vi "New Three.vi"() -> ()   [LabVIEW 2015]
doc: "This example VI shows how to convert string data elements to numeric elements so it can be graphed and displayed on an XY Graph."
uses:
  <instrlib>/Keithley 27XX/Public/Configure/Measurement Specific/Configure Thermocouple.vi
  <instrlib>/Keithley 27XX/Keithley 27XX.lvlib
panel:
  out "Voltage 2":dbl(graph)
  out "Voltage 1":dbl(graph)
  out "Temperature Ch 1":dbl(graph)
  out "Temperature Ch 2":dbl(graph)
  out "appended array":dbl[](array[numeric])
  out "Iteration":i32
  out "x-y":dbl
  in  "Pause/Continue":bool
  out "error out 2425":errorcluster
  in  "range":i32
  in  "function":i32(slide)
  in  "error in (no error) 2":errorcluster
  in  "reset device":u16(slide)=1
  in  "id query":u16(slide)=1
  in  "resource name":string="GPIB0::20::INSTR"
  out "Temp Ch 4":dbl
  out "Temp Ch 3":dbl
  out "Temp Ch 2":dbl
  out "Temp Ch 1":dbl
  out "Voltage Ch 1":dbl
  out "Voltage Ch 2":dbl
  in  "stop":bool
  in  "Number of channels 2":i32=2
  in  "Function (0: DC Voltage)":u16(ring) items=["DC Voltage", "AC Voltage", "DC Current", "AC Current", "Resistance", "Four-Wire Resistance", "Temperature (C)", "Frequency", "Period", "Continuity"]
  in  "Channel List (101) 2":string="101:102"
  in  "Serial Configuration 2":T1={"Baud Rate (9600)"=9600, "Flow Control (1: XON/XOFF)"=1, "Termination Char (0:CR)"=0} {"Termination Char (0:CR)" items=["CR", "LF", "CRLF (Do not use)", "LFCR (Do not use)"]; "Flow Control (1: XON/XOFF)" items=["None", "XON/XOFF", "RTS/CTS (2701 Only)", "XON/XOFF & RTS/CTS (2701 Only)"]; "Baud Rate (9600)" items=["300"=300, "600"=600, "1200"=1200, "2400"=2400, "4800"=4800, "9600"=9600, "19.2k"=19200, "38.4k (2701 Only)"=38400, "57.6k (2701 Only)"=57600, "115.2k (2701 Only)"=115200]}
  in  "Keithley VISA resource name 2":refnum<visa-resource-name>="GPIB0::19::INSTR"
  in  "Enable Open Detector? (False)":bool=TRUE
  in  "Simulated Reference Temperature (23 deg C)":dbl=23.0
  in  "Reference Junction Type (1: Internal)":u16(ring)=1 items=["Simulated", "Internal", "External"]
  in  "Thermocouple Type (1: K)":u16(ring)=1 items=["J", "K", "T", "E", "R", "S", "B", "N"]
  in  "Number of channels":i32=4
  in  "Function (6: Temp)":u16(ring)=6 items=["DC Voltage", "AC Voltage", "DC Current", "AC Current", "Resistance", "Four-Wire Resistance", "Temperature (C)", "Frequency", "Period", "Continuity"]
  in  "Channel List (101)":string="101"
  in  "Serial Configuration":T1={"Baud Rate (9600)"=9600, "Flow Control (1: XON/XOFF)"=1, "Termination Char (0:CR)"=0} {"Termination Char (0:CR)" items=["CR", "LF", "CRLF (Do not use)", "LFCR (Do not use)"]; "Flow Control (1: XON/XOFF)" items=["None", "XON/XOFF", "RTS/CTS (2701 Only)", "XON/XOFF & RTS/CTS (2701 Only)"]; "Baud Rate (9600)" items=["300"=300, "600"=600, "1200"=1200, "2400"=2400, "4800"=4800, "9600"=9600, "19.2k"=19200, "38.4k (2701 Only)"=38400, "57.6k (2701 Only)"=57600, "115.2k (2701 Only)"=115200]}
  in  "Keithley VISA resource name":refnum<visa-resource-name>="GPIB0::19::INSTR"
  # "2700 Temp INIT"
  # "Keithley 2425 INIT"
  # "2700 Voltage INIT"
  # "File INIT"
  # "Operations"
  # "Only 4 Ch implemented"
  # "Data"
  # "Loop 1"
  # "Loop 2"
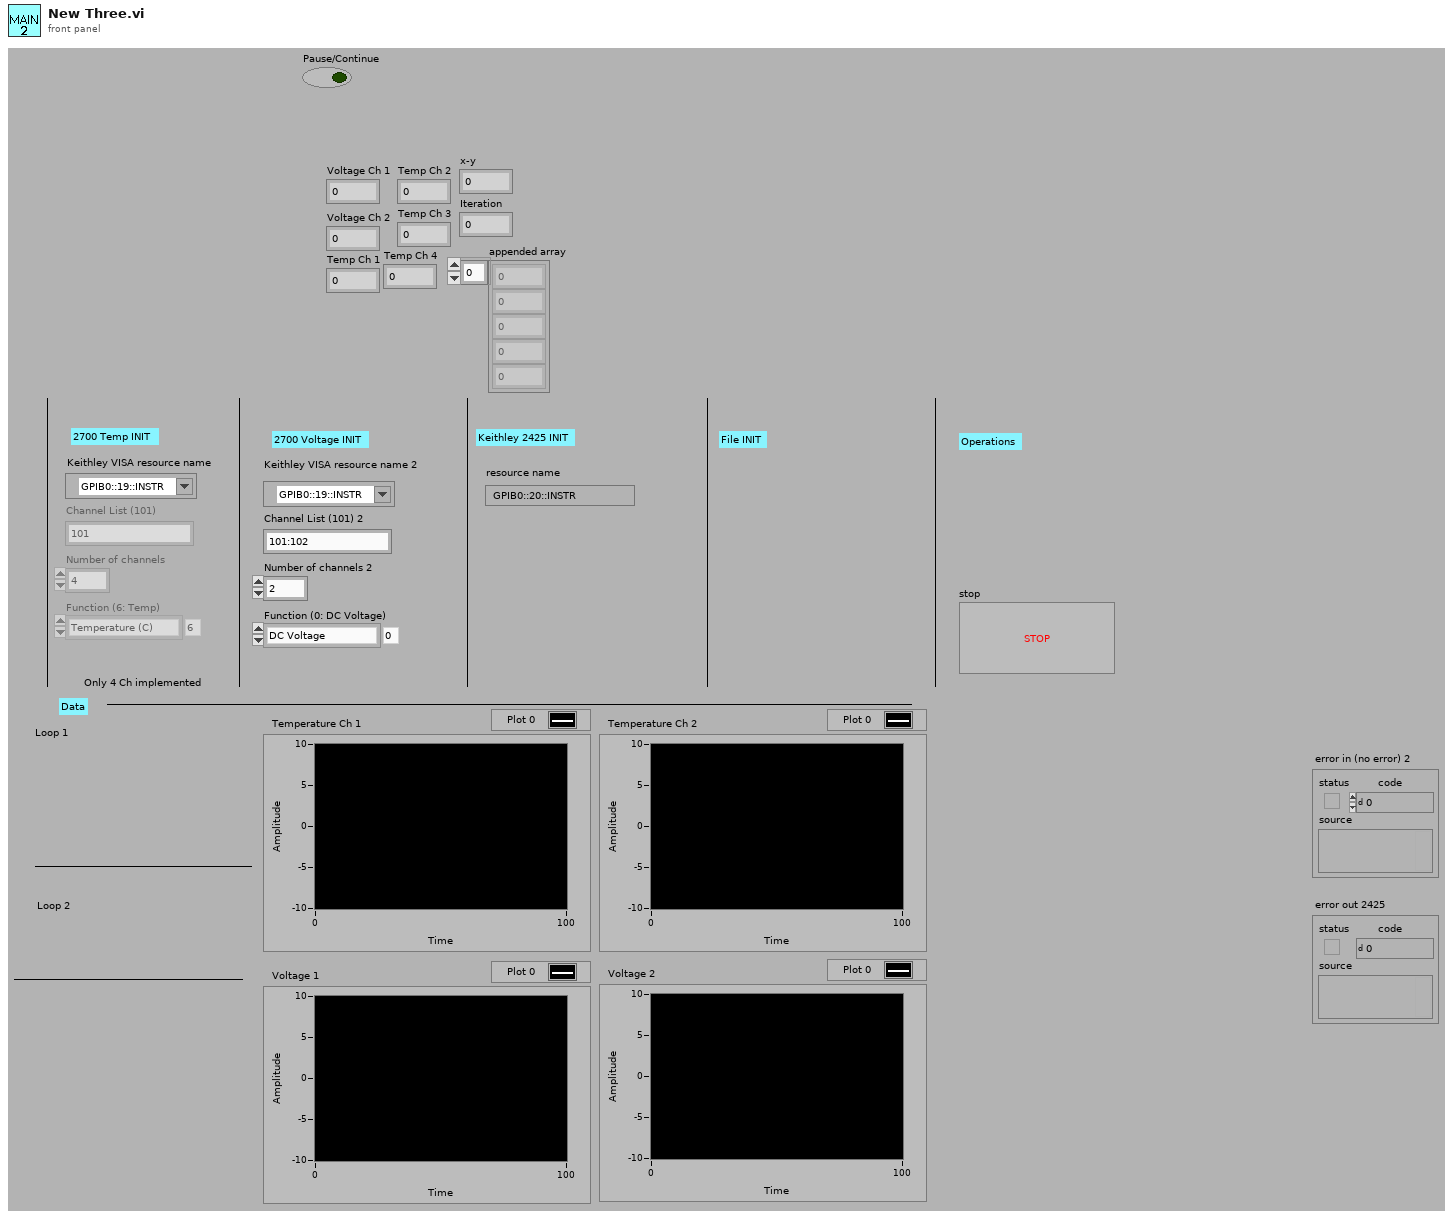
[diagram p1: front panel]
types:
  T1 = cluster{"Baud Rate (9600)":u32, "Flow Control (1: XON/XOFF)":u16, "Termination Char (0:CR)":u16}
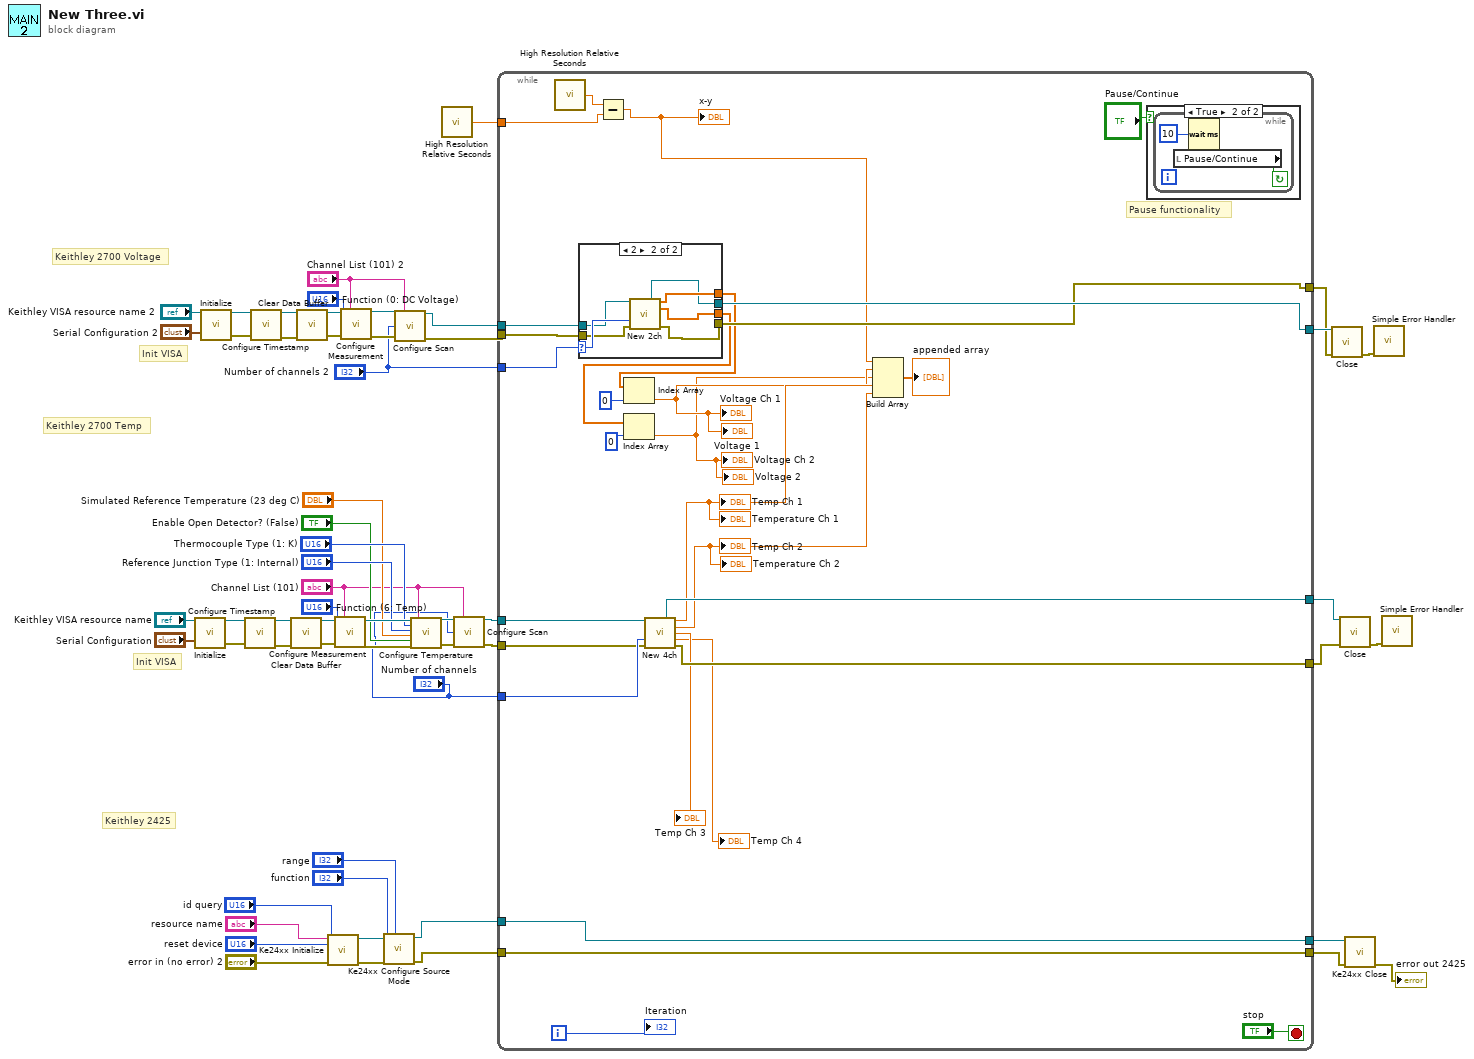
[diagram p0: block diagram]
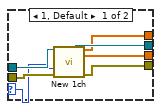
[diagram p3: hidden frame]
diagram:
  # "Keithley 2425"
  # "Keithley 2700 Voltage"
  # "Init VISA"
  # "Keithley 2700 Temp"
  # "Init VISA"
  n1 = call <instrlib>:"Initialize.vi"("VISA resource name"="Keithley VISA resource name", "Serial Configuration"="Serial Configuration") -> ("VISA resource name out"=w54:refnum<visa-resource-name>, "error out"=w53:errorcluster)  [unwired: 12 in]
  n2 = call <instrlib>:"Initialize.vi"("VISA resource name"="Keithley VISA resource name 2", "Serial Configuration"="Serial Configuration 2") -> ("VISA resource name out"=w36:refnum<visa-resource-name>, "error out"=w35:errorcluster)  [unwired: 12 in]
  n3 = call <instrlib>:"Configure Timestamp.vi"("VISA resource name"=w54, "error in (no error)"=w53) -> ("VISA resource name out"=w51:refnum<visa-resource-name>, "error out"=w50:errorcluster)  [unwired: 12 in]
  n4 = call <instrlib>:"Configure Timestamp.vi"("VISA resource name"=w36, "error in (no error)"=w35) -> ("VISA resource name out"=w33:refnum<visa-resource-name>, "error out"=w32:errorcluster)  [unwired: 12 in]
  n5 = call <instrlib>:"Clear Data Buffer.vi"("VISA resource name"=w51, "error in (no error)"=w50) -> ("VISA resource name out"=w49:refnum<visa-resource-name>, "error out"=w52:errorcluster)  [unwired: 12 in]
  n6 = call <instrlib>:"Clear Data Buffer.vi"("VISA resource name"=w33, "error in (no error)"=w32) -> ("VISA resource name out"=w31:refnum<visa-resource-name>, "error out"=w34:errorcluster)  [unwired: 12 in]
  n7 = call <instrlib>:"Ke24xx Initialize.vi"("error in (no error)"="error in (no error) 2", "reset device"="reset device", "id query"="id query", "resource name"="resource name") -> ("error out"=w9:errorcluster, "instrument handle out"=w10:refnum<visa-resource-name>)  [unwired: 5 in, 1 out]
  n8 = call <instrlib>:"Configure Measurement.vi"("VISA resource name"=w49, "Scan List (Empty)"="Channel List (101)", "Function (0: DC Voltage)"="Function (6: Temp)", "error in (no error)"=w52) -> ("VISA resource name out"=w47:refnum<visa-resource-name>, "error out"=w44:errorcluster)  [unwired: 10 in]
  n9 = call <instrlib>:"Configure Measurement.vi"("VISA resource name"=w31, "Scan List (Empty)"="Channel List (101) 2", "Function (0: DC Voltage)"="Function (0: DC Voltage)", "error in (no error)"=w34) -> ("VISA resource name out"=w29:refnum<visa-resource-name>, "error out"=w28:errorcluster)  [unwired: 10 in]
  n10 = call <instrlib>:"Ke24xx Configure Source Mode.vi"("range"="range", "error in (no error)"=w9, "function"="function", "instrument handle"=w10) -> ("error out"=w4:errorcluster, "instrument handle out"=w3:refnum<visa-resource-name>)  [unwired: 5 in, 1 out]
  n11 = call <instrlib>:"Configure Scan.vi"("VISA resource name"=w29, "Channel List (101:110)"="Channel List (101) 2", "Sample Count (100)"="Number of channels 2", "error in (no error)"=w28) -> ("VISA resource name out"=w26:refnum<visa-resource-name>, "error out"=w25:errorcluster)  [unwired: 10 in]
  n12 = call-poly <instrlib>:"Configure Temperature.vi"("VISA resource name"=w47, "Thermocouple Type (1: K)"="Thermocouple Type (1: K)", "Reference Junction Type (0: Simulated)"="Reference Junction Type (1: Internal)", "Simulated Reference Temperature (23 deg C)"="Simulated Reference Temperature (23 deg C)", "Enable Open Detector? (False)"="Enable Open Detector? (False)", "error in (no error)"=w44, "Scan List (Empty)"="Channel List (101)") -> ("VISA resource name out"=w46:refnum<visa-resource-name>, "error out"=w45:errorcluster)  [unwired: 11 in]
  n13 = call <vilib>:"High Resolution Relative Seconds.vi"() -> ("relative seconds"=w1:dbl)
  n14 = call <instrlib>:"Configure Scan.vi"("VISA resource name"=w46, "Channel List (101:110)"="Channel List (101)", "Sample Count (100)"="Number of channels", "error in (no error)"=w45) -> ("VISA resource name out"=w24:refnum<visa-resource-name>, "error out"=w23:errorcluster)  [unwired: 10 in]
  n15 = while {
    tunnel: w26 -> [w84]
    tunnel: w25 -> [w83]
    tunnel: w24 -> [w75]
    tunnel: w23 -> [w73]
    tunnel: "Number of channels" -> [w74]
    tunnel: "Number of channels 2" -> [w82]
    tunnel: [w81] -> w18
    tunnel: [w80] -> w17
    tunnel: [w71] -> w16
    tunnel: [w72] -> w15
    tunnel: [w68] -> w5
    tunnel: w4 -> [w68]
    tunnel: w3 -> [w67]
    tunnel: [w67] -> w2
    tunnel: w1 -> [w64]
    i -> [w63]
    stop <- "stop" stop-if-true
    # "Pause functionality"
    n16 = call <vilib>:"High Resolution Relative Seconds.vi"() -> ("relative seconds"=w65:dbl)
    n17 = case shown="2" w82 {
      selector: w82 -> [w92 w101]
      tunnel: w84 -> [w94 w99]
      tunnel: w83 -> [w93 w100]
      tunnel: [w91 w95] -> w81
      tunnel: [w90 w97] -> w80
      tunnel: [w89 w98] -> w76
      tunnel: [w88 w96] -> w78
      frame 1, Default {
        n18 = call "New 1ch.vi"("VISA resource name out"=w94, "Number of channels"=w92, "error out"=w93) -> ("VISA resource name out 2"=w91:refnum<visa-resource-name>, "Array 2"=w89:dbl[], "Array"=w88:dbl[], "error out 2"=w90:errorcluster)  [unwired: 9 in]
      }
      frame 2 {
        n19 = call "New 2ch.vi"("VISA resource name out"=w99, "Number of channels"=w101, "error out"=w100) -> ("VISA resource name out 2"=w95:refnum<visa-resource-name>, "Array 2"=w98:dbl[], "Array"=w96:dbl[], "error out 2"=w97:errorcluster)  [unwired: 9 in]
      }
    }
    n20 = Subtract(x=w65, y=w64) -> (x-y=w62:dbl)
    "x-y" <- w62
    n21 = Index Array(array=w76, index=0) -> (element=w58:dbl)
    "Voltage Ch 1" <- w58
    "Voltage 1" <- w58
    n22 = Index Array(array=w78, index=0) -> (element=w57:dbl)
    "Voltage Ch 2" <- w57
    "Voltage 2" <- w57
    n23 = call "New 4ch.vi"("VISA resource name out"=w75, "Number of channels"=w74, "error out"=w73) -> ("VISA resource name out 2"=w72:refnum<visa-resource-name>, "element"=w59:dbl, "element 2"=w60:dbl, "element 3"=→"Temp Ch 3":dbl, "element 4"=→"Temp Ch 4":dbl, "error out 2"=w71:errorcluster)  [unwired: 7 in]
    "Temp Ch 1" <- w59
    "Temp Ch 2" <- w60
    "Temperature Ch 2" <- w60
    "Temperature Ch 1" <- w59
    n24 = Build Array(w62, w58, w57, w59, w60) -> (→"appended array":dbl[])
    n25 = case shown="True" "Pause/Continue" {
      frame False {
      }
      frame True {
        n26 = while {
          stop <- w87 continue-if-true
          n27 = local read "Pause/Continue"() -> (w87:bool)
          n28 = Wait (ms)(milliseconds to wait=u32 10) -> ()  [unwired: 1 out]
        }
      }
    }
    "Iteration" <- w63
  }
  n29 = call <instrlib>:"Close.vi"("VISA resource name"=w18, "error in (no error)"=w17) -> ("error out"=w20:errorcluster)  [unwired: 13 in]
  n30 = call <instrlib>:"Close.vi"("VISA resource name"=w15, "error in (no error)"=w16) -> ("error out"=w19:errorcluster)  [unwired: 13 in]
  n31 = call <instrlib>:"Ke24xx Close.vi"("error in (no error)"=w5, "instrument handle"=w2) -> ("error out"=→"error out 2425":errorcluster)  [unwired: 8 in, 1 out]
  n32 = call <vilib>:"Simple Error Handler.vi"("error in (no error)"=w20) -> ()  [unwired: 4 in, 5 out]
  n33 = call <vilib>:"Simple Error Handler.vi"("error in (no error)"=w19) -> ()  [unwired: 4 in, 5 out]
